vi "UTIL Progress Bar Update Current.vi"(8 "error in (no error)":errorcluster, 10 "Current":i32, 11 "reference in":refnum<vi>) -> (0 "error out":errorcluster, 3 "reference out":refnum<vi>)   [LabVIEW 2019]
doc: "10/01/2010\n\nNational Analytics (TLE)\n\nUpdate the current value of the progress bar."
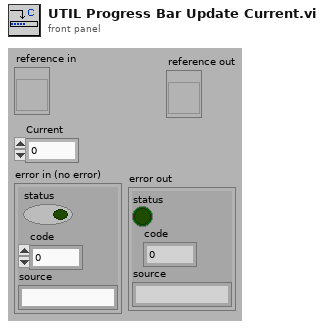
[diagram p1: front panel]
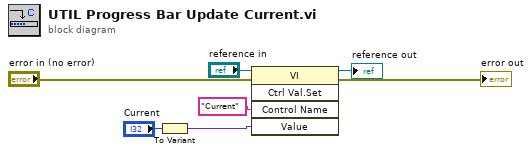
[diagram p0: block diagram]
diagram:
  n1 = To Variant(anything="Current") -> (Variant=w1:variant)
  n2 = invoke class="VI" method="Ctrl Val.Set"(reference="reference in", error in="error in (no error)", "Control Name"="Current", "Value"=w1) -> (reference out=→"reference out":refnum<vi>, error out=→"error out":errorcluster)  [unwired: 1 in, 3 out]
